vi "Write AutoSizeColumnsMode.vi"(8 "error in (no error)":errorcluster, 10 "AutoSizeColumnsMode":i32(ring)=10 items=["None"=1, "ColumnHeader"=2, "AllCellsExceptHeader"=4, "AllCells"=6, "DisplayedCellsExceptHeader"=8, "DisplayedCells"=10, "Fill"=16], 11 "DataGridView in":refnum<class "DataGridView.lvclass">) -> (0 "error out":errorcluster, 3 "DataGridView out":refnum<class "DataGridView.lvclass">)   [LabVIEW 2013, in "DataGrid.lvlib" / "DataGridView.lvclass"]
uses:
  DataGridView.lvclass
  DataGridView.lvclass/DataGridView.ctl
  System.Windows.Forms
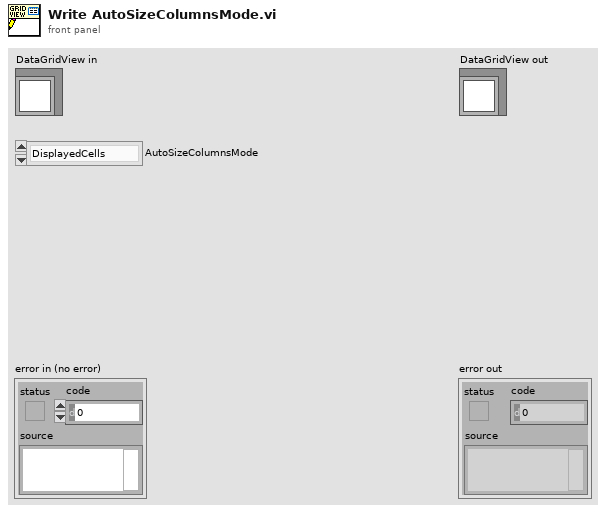
[diagram p1: front panel]
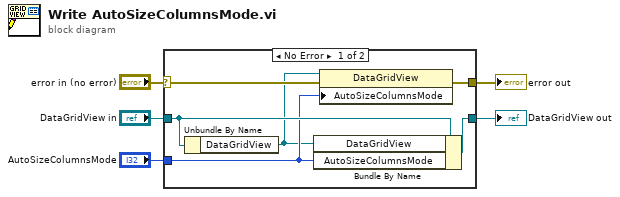
[diagram p0: block diagram]
diagram:
  n1 = case shown="No Error" "error in (no error)" {
    selector: "error in (no error)" -> [w8 w12]
    tunnel: [w7 w12] -> w4
    tunnel: [w11 w13] -> w2
    tunnel: "DataGridView in" -> [w10 w13]
    tunnel: "AutoSizeColumnsMode" -> [w9 _]
    frame No Error {
      n2 = Unbundle By Name(w10) -> ("DataGridView"=w6:refnum<k24>)
      n3 = Bundle By Name(cluster=w10, "DataGridView"=w6, "AutoSizeColumnsMode"=w9) -> (w11:refnum<class "DataGridView.lvclass">)
      n4 = property class="DataGridView"(reference=w6, error in=w8, "AutoSizeColumnsMode"=w9) -> (error out=w7:errorcluster)  [unwired: 1 out]
    }
    frame Error {
    }
  }
  "error out" <- w4
  "DataGridView out" <- w2
